vi "MIMIC Commands Rev 2.vi"(6 "MIMIC HOST COMMAND":T2(ring)=enum."Read Serial Number", 8 "Input String Data Array":string[](array[string])=["1"], 9 "HWHSflag":bool, 10 "wait (ms)":u32=500, 11 "VISA resource name":refnum<visa-resource-name>="COM5") -> (0 "error out":errorcluster={"status"=FALSE, "code"=1073676294, "source"="VISA Read in MIMIC RecvCommand.vi->MIMIC Commands Rev 2.vi"}, 1 "Receive_buffer":u8[](array[numeric]), 2 "Receive_Unpacked_Data":T1)   [LabVIEW 2014]
panel:
  out "Array":u8[](array[numeric])
  out "TimeToDecode":u16
  out "VISA resource name OUT":refnum<visa-resource-name>="COM5"
  out "hex integer string":string[](array[string])=["4", "D0", "0", "0", "FF", "2C"]
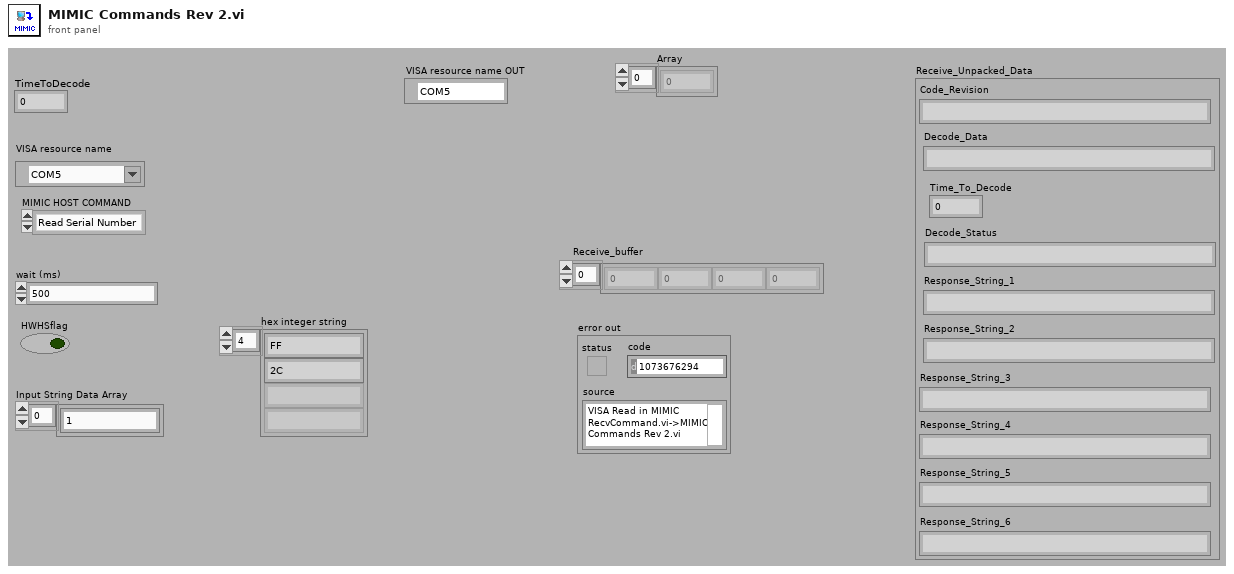
[diagram p1: front panel]
types:
  T1 = cluster{"Code_Revision":string, "Decode_Data":string, "Decode_Status":string, "Response_String_1":string, "Response_String_2":string, "Response_String_3":string, "Response_String_4":string, "Response_String_5":string, "Response_String_6":string, "Time_To_Decode":u16}
  T2 = enum16{"Enter FAT", "Beeper Control", "LED Off", "LED On", "Image Mode", "Start Session", "Stop Session", "Change Buadrate", "Auto Exposure", "Set Manual Exposure", "Read BT Address", "Store BT Address", "Pairing Command", "Query Paired Address", "Pairing Status", "Un-Pairing", "Set Illumination", "Trigger", "Set Defaults", "Imager Time To Decode Test", "Battery Off", "Battery Charge Control", "Read Battery Voltage", "Read Battery Temperature", "Software Version", "Store Feature Set", "Read Feature Set", "Store Model Number", "Read Model Number", "Store Manufacturing Date", "Read Manufacturing Date", "Store Service Date", "Read Service Date", "Store Serial Number", "Read Serial Number", "Exit FAT"}
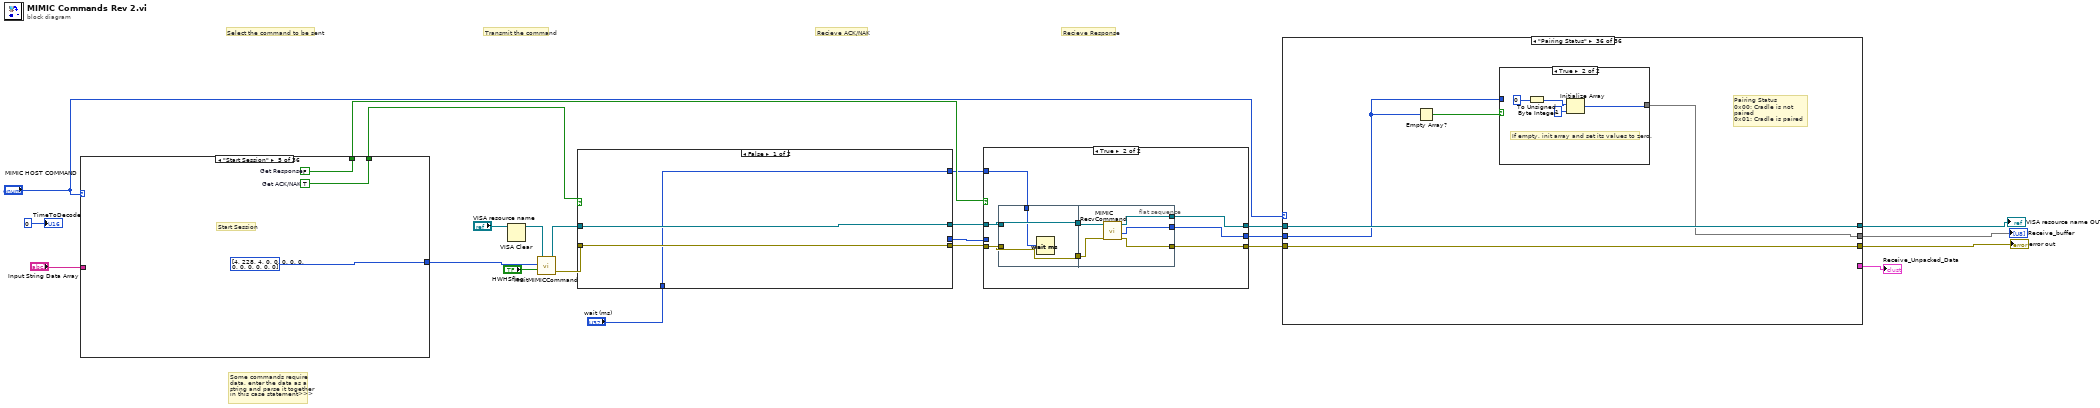
[diagram p0: block diagram]
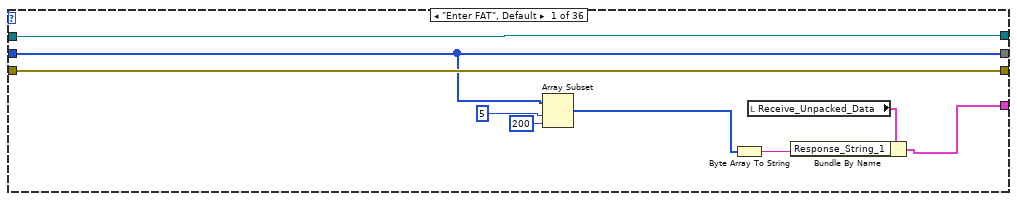
[diagram p2: hidden frame]
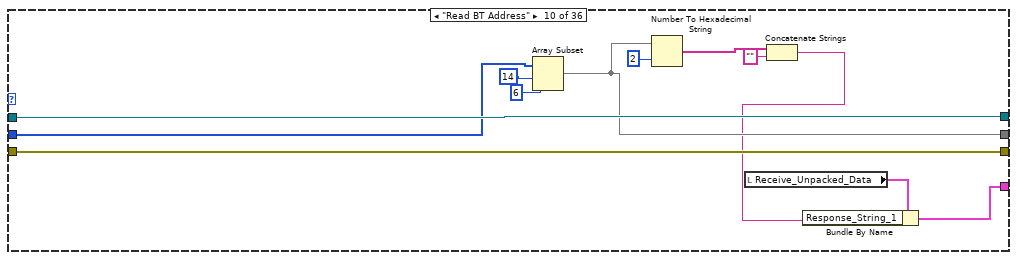
[diagram p11: hidden frame]
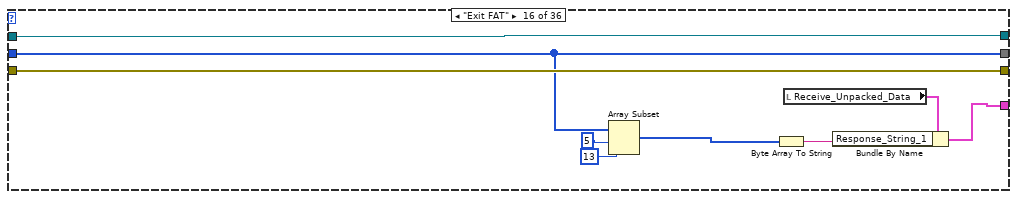
[diagram p17: hidden frame]
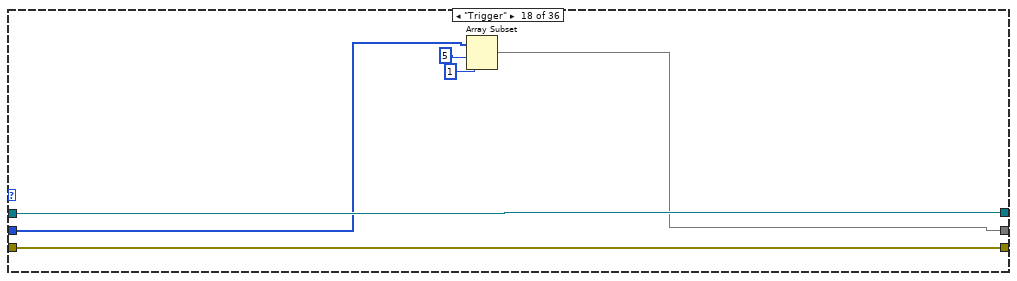
[diagram p19: hidden frame]
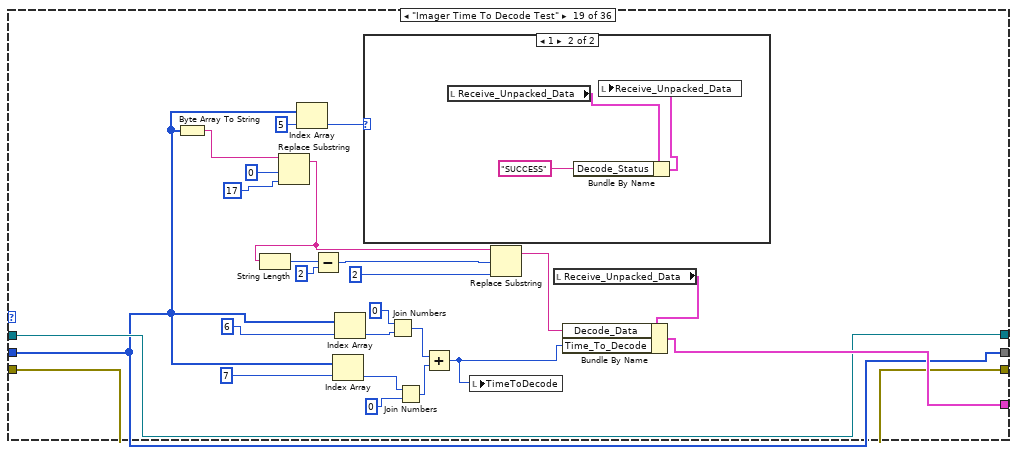
[diagram p20: hidden frame]
diagram:
  # "Transmit the command"
  # "Recieve Response"
  # "Recieve ACK/NAK"
  # "Select the command to be sent"
  # "Some commands require\ndata, enter the data as a\nstring and parse it together\nin this case statement>>>"
  n1 = case shown="\"Start Session\"" "MIMIC HOST COMMAND" {
    tunnel: "Input String Data Array" -> [w32 w33 _ w44 _ _ _ w62 w78 w88 w101 _ _ _ _ _ w125 _ _ _ w145 _ _ _ w161 _ w173 _ _ _ w199 _ w211 _ _ _]
    tunnel: [w26 w37 u8[] [5, 161, 4, 128, 16, 0, 0, 0, 0, 0, 0, 0, 0, 0] w45 u8[] [4, 228, 4, 0, 0, 0, 0, 0, 0, 0, 0, 0, 0, 0] u8[] [4, 228, 4, 0, 0, 0, 0, 0, 0, 0, 0, 0, 0, 0] u8[] [7, 215, 4, 0, 4, 11, 0, 255, 15, 0, 0, 0, 0, 0] w63 w72 w86 w100 u8[] [16, 161, 4, 128, 16, 0, 0, 0, 0, 0, 0, 0, 0, 0] u8[] [5, 161, 4, 128, 16, 0, 0, 0, 0, 0, 0, 0, 0, 0] u8[] [4, 200, 4, 128, 0, 0, 0, 0, 0, 0, 0, 0, 0, 0] u8[] [5, 161, 4, 128, 25, 0, 0, 0, 0, 0, 0, 0, 0, 0] u8[] [7, 161, 4, 128, 66, 2, 29, 0, 0, 0, 0, 0, 0, 0] w124 u8[] [6, 161, 4, 128, 45, 2, 0, 0, 0, 0, 0, 0, 0, 0] u8[] [7, 161, 4, 128, 48, 19, 136, 0, 0, 0, 0, 0, 0, 0] u8[] [5, 161, 4, 128, 60, 0, 0, 0, 0, 0, 0, 0, 0, 0] w144 u8[] [7, 161, 4, 128, 66, 117, 48, 0, 0, 0, 0, 0, 0, 0] u8[] [7, 161, 4, 128, 66, 117, 49, 0, 0, 0, 0, 0, 0, 0] u8[] [7, 161, 4, 128, 66, 78, 41, 0, 0, 0, 0, 0, 0, 0] w165 u8[] [7, 161, 4, 128, 66, 2, 194, 0, 0, 0, 0, 0, 0, 0] w178 u8[] [7, 161, 4, 128, 66, 2, 21, 0, 0, 0, 0, 0, 0, 0] w192 u8[] [7, 161, 4, 128, 66, 2, 23, 0, 0, 0, 0, 0, 0, 0] w204 u8[] [7, 161, 4, 128, 66, 2, 24, 0, 0, 0, 0, 0, 0, 0] w216 u8[] [7, 161, 4, 128, 66, 2, 22, 0, 0, 0, 0, 0, 0, 0] u8[] [5, 161, 4, 128, 54, 254, 160, 0, 0, 0, 0, 0, 0, 0] u8[] [5, 161, 4, 128, 84, 0, 0, 0, 0, 0, 0, 0, 0, 0]] -> w18
    tunnel: [w25 w35 w42 w46 w54 w57 w59 w64 w79 w89 w107 w110 w112 w115 w119 w123 w127 w134 w138 w141 w142 w153 w156 w158 w168 w171 w177 w182 w191 w196 w203 w207 w214 w219 w223 w227] -> w20
    tunnel: [w24 w36 w41 w47 w55 w58 w60 w65 w80 w90 w108 w111 w113 w116 w118 w122 w126 w135 w137 w140 w143 w152 w155 w157 w167 w170 w176 w183 w190 w195 w202 w208 w215 w220 w222 w226] -> w22
    frame "LED On" {
      w25 = FALSE  # Get Response
      w24 = TRUE  # Get ACK/NAK
      # "LED data Byte"
      n2 = Index Array(array=w32, index=0) -> (element=w31:string)
      n3 = Decimal String To Number(string=w31) -> (number=w30:i32)  [unwired: 2 in, 1 out]
      n4 = Replace Array Subset(array=u8[] [5, 231, 4, 128, 1, 0, 0, 0, 0, 0, 0, 0, 0, 0], new element=w30, index=4) -> (w26:u8[])
    }
    frame "Beeper Control" {
      w35 = FALSE  # Get Response
      w36 = FALSE  # Get ACK/NAK
      # "Beeper data Byte"
      n5 = Decimal String To Number(string=w33, offset=0) -> (number=w40:i32[])  [unwired: 1 in, 1 out]
      n6 = Replace Array Subset(array=u8[] [5, 230, 4, 128, 0, 0, 0, 0, 0, 0, 0, 0, 0, 0], new element=w40, index=4) -> (w37:u8[])
    }
    frame "Enter FAT" {
      w42 = TRUE  # Get Response
      w41 = TRUE  # Get ACK/NAK
      # "Enter FAT command:\n0x05:0xA1:0x40:0x80:0x10"
    }
    frame "Image Mode" {
      w46 = FALSE  # Get Response
      w47 = TRUE  # Get ACK/NAK
      # "Image Mode Byte:\n00: Decode\n01: SnapShot\n02: Video\n03: Last Decode\n04: las No Decode"
      n7 = Index Array(array=w44, index=0) -> (element=w52:string)
      n8 = Decimal String To Number(string=w52) -> (number=w51:i32)  [unwired: 2 in, 1 out]
      n9 = Replace Array Subset(array=u8[] [5, 247, 4, 128, 0, 0, 0, 0, 0, 0, 0, 0, 0, 0], new element=w51, index=4) -> (w45:u8[])
    }
    frame "Start Session" {
      w54 = FALSE  # Get Response
      w55 = TRUE  # Get ACK/NAK
      # "Start Session"
    }
    frame "Stop Session" {
      w57 = FALSE  # Get Response
      w58 = TRUE  # Get ACK/NAK
      # "Start Session"
    }
    frame "Change Buadrate" {
      w59 = FALSE  # Get Response
      w60 = FALSE  # Get ACK/NAK
      # "Enter FAT command:\n06: 9600\n08: 38400\n0A: 57600\n0B:115200\n0C:230400"
    }
    frame "Auto Exposure" {
      w64 = FALSE  # Get Response
      w65 = TRUE  # Get ACK/NAK
      # "Auto Exposure:\n00:Disabled\n01: Enabled"
      n10 = Index Array(array=w62, index=0) -> (element=w70:string)
      n11 = Decimal String To Number(string=w70) -> (number=w69:i32)  [unwired: 2 in, 1 out]
      n12 = Replace Array Subset(array=u8[] [8, 198, 4, 0, 255, 240, 41, 0, 0, 0, 0, 0, 0, 0], new element=w69, index=7) -> (w63:u8[])
    }
    frame "Set Manual Exposure" {
      w79 = FALSE  # Get Response
      w80 = TRUE  # Get ACK/NAK
      # "Image Mode Byte:\n00: Decode\n01: SnapShot\n02: Video\n03: Last Decode\n04: las No Decode"
      n13 = Index Array(array=w78, index=0) -> (element=w84:string)
      n14 = Decimal String To Number(string=w84, default (0L)=u16 0 ("default (0 I32)")) -> (number=w77:u16)  [unwired: 1 in, 1 out]
      n15 = Split Number(x=w77) -> (hi(x)=w75:u8, lo(x)=w74:u8)
      n16 = Replace Array Subset(array=u8[] [10, 198, 4, 0, 255, 244, 241, 55, 0, 0, 0, 0, 0, 0], new element=w75, index=8) -> (w71:u8[])
      n17 = Replace Array Subset(array=w71, new element=w74, index=9) -> (w72:u8[])
    }
    frame "Store BT Address" {
      w89 = FALSE  # Get Response
      w90 = TRUE  # Get ACK/NAK
      # "Store BT command:\n0x16, 0xA1, 0x04, 0x80, 0x45, 0x02, 0x1D, 0x41, 0x07, 0x42, 0x00, 0x06, 0x00, 0x00, \n\t\t\t\t\t\t\t\t\t\t0x00, 0x00, 0x00, 0x00, 0x00, 0x00,0x00, 0x00, 0xFF, 0xFF};"
      n18 = for {
        N: 6 -> [_]
        tunnel: w88 -> [w99]
        tunnel: [w94] -> w86
        i -> [w96]
        n19 = Index Array(array=w99, index=w96) -> (element=w93:string)
        n20 = Add(x=14 ("index"), y=w96) -> (x+y=w97:i32)
        n21 = Hexadecimal String To Number(string=w93, offset=0) -> (number=w91:u32)  [unwired: 1 in, 1 out]
        n22 = local read "Array"() -> (w95:u8[])
        n23 = Replace Array Subset(array=w95, new element=w91, index=w97) -> (w94:u8[])
        n24 = local write "Array"(w94) -> ()
      }
      "Array" <- u8[] [22, 161, 4, 128, 69, 2, 29, 65, 7, 66, 0, 6, 0, 0, 0, 0, 0, 0, 0, 0, 255, 255, 255, 0, 0, 0]
    }
    frame "Pairing Command" {
      w107 = TRUE  # Get Response
      w108 = FALSE  # Get ACK/NAK
      # "Pairing  command:\n10 9E 04 80 00 00 02 03 06 08  01 0B 03 00 0F 0F FE 8E"
      n25 = Index Array(array=w101, index=0) -> (element=w105:string)
      n26 = String To Byte Array(string=w105) -> (unsigned byte array=w103:u8[])
      n27 = Replace Array Subset(array=u8[] [16, 158, 4, 128, 0, 0, 0, 0, 0, 8, 1, 11, 3, 0, 15, 15], new element=w103, index=4) -> (w100:u8[])
    }
    frame "Un-Pairing" {
      w110 = TRUE  # Get Response
      w111 = FALSE  # Get ACK/NAK
      # "Enter FAT command:\n0x05:0xA1:0x40:0x80:0x10"
    }
    frame "Set Illumination" {
      w112 = TRUE  # Get Response
      w113 = FALSE  # Get ACK/NAK
      # "Enter FAT command:\n0x05:0xA1:0x40:0x80:0x10"
    }
    frame "Set Defaults" {
      w115 = FALSE  # Get Response
      w116 = TRUE  # Get ACK/NAK
    }
    frame "Exit FAT" {
      w119 = TRUE  # Get Response
      w118 = TRUE  # Get ACK/NAK
    }
    frame "Read BT Address" {
      w123 = TRUE  # Get Response
      w122 = FALSE  # Get ACK/NAK
    }
    frame "LED Off" {
      w127 = FALSE  # Get Response
      w126 = TRUE  # Get ACK/NAK
      # "LED data Byte"
      n28 = Index Array(array=w125, index=0) -> (element=w132:string)
      n29 = Decimal String To Number(string=w132) -> (number=w131:i32)  [unwired: 2 in, 1 out]
      n30 = Replace Array Subset(array=u8[] [5, 232, 4, 128, 1, 0, 0, 0, 0, 0, 0, 0, 0, 0], new element=w131, index=4) -> (w124:u8[])
    }
    frame "Trigger" {
      w134 = TRUE  # Get Response
      w135 = TRUE  # Get ACK/NAK
    }
    frame "Imager Time To Decode Test" {
      w138 = TRUE  # Get Response
      w137 = TRUE  # Get ACK/NAK
      # "Start Session"
    }
    frame "Battery Off" {
      w141 = FALSE  # Get Response
      w140 = TRUE  # Get ACK/NAK
      # "Enter FAT command:\n0x05:0xA1:0x40:0x80:0x10"
    }
    frame "Battery Charge Control" {
      w142 = FALSE  # Get Response
      w143 = TRUE  # Get ACK/NAK
      # "Battery Charge\n0x06, 0xA1, 0x04, 0x80, 0x3D\n0x00: Disable charging of battery\n0x01: Enable charging of battery\n0x02: Enable Slow charge (Hammer)"
      n31 = Index Array(array=w145, index=0) -> (element=w150:string)
      n32 = Decimal String To Number(string=w150) -> (number=w149:i32)  [unwired: 2 in, 1 out]
      n33 = Replace Array Subset(array=u8[] [6, 161, 4, 128, 61, 0, 0, 0, 0, 0, 0, 0, 0, 0], new element=w149, index=5) -> (w144:u8[])
    }
    frame "Read Battery Voltage" {
      w153 = TRUE  # Get Response
      w152 = FALSE  # Get ACK/NAK
      # "Read Battery Voltage command:\n0x07:0xA1:0x04:0x80:0x42:0x75:0x30"
    }
    frame "Read Battery Temperature" {
      w156 = TRUE  # Get Response
      w155 = FALSE  # Get ACK/NAK
      # "Read Battery Temperature command:\n0x07:0xA1:0x04:0x80:0x42:0x75:0x31"
    }
    frame "Software Version" {
      w158 = TRUE  # Get Response
      w157 = TRUE  # Get ACK/NAK
      # "Software Version command:\n\"0x07, 0xA1, 0x04, 0x80, 0x42, 0x4E, 0x29,\""
    }
    frame "Store Feature Set" {
      w168 = FALSE  # Get Response
      w167 = TRUE  # Get ACK/NAK
      # "Store Feature Set command:\n\"0x0A, 0xA1, 0x04, 0x80, 0x45, 0x02, 0xC2, 0x42, 0x07,\n0xFF,//Feature Set Value \n0x00, 0x00}; //checksum\""
      n34 = Index Array(array=w161, index=0) -> (element=w163:string)
      n35 = String To Byte Array(string=w163) -> (unsigned byte array=w160:u8[])
      n36 = Replace Array Subset(array=u8[] [10, 161, 4, 128, 69, 2, 194, 66, 7, 0, 0, 0, 0, 0], new element=w160, index=9) -> (w165:u8[])
    }
    frame "Read Feature Set" {
      w171 = TRUE  # Get Response
      w170 = FALSE  # Get ACK/NAK
      # "Read Feature Set command:\n0x07, 0xA1, 0x04, 0x80, 0x42, 0x02, 0xC2,"
    }
    frame "Store Model Number" {
      w177 = FALSE  # Get Response
      w176 = TRUE  # Get ACK/NAK
      # "StoreModel Number command:\n0x20, 0xA1, 0x04, 0x80, 0x45, 0x02, 0x15, 0x53, 0x07, 0x00, 0x12, 0x00, 0x00,\n\t\t\t\t\t\t\t\t\t\t0x00, 0x00, 0x00, 0x00, 0x00, 0x00, 0x00, 0x00, 0x00,\n\t\t\t\t\t\t\t\t\t\t0x00, 0x00, 0x00, 0x00, 0x00, 0x00, 0x00, 0x00, 0x00,\n\t\t\t\t\t\t\t\t\t\t0x00"
      n37 = Index Array(array=w173, index=0) -> (element=w174:string)
      n38 = String To Byte Array(string=w174) -> (unsigned byte array=w175:u8[])
      n39 = Replace Array Subset(array=u8[] [32, 161, 4, 128, 69, 2, 21, 83, 7, 0, 18, 0, 0, 0, 0, 0, 0, 0, 0, 0, 0, 0, 0, 0, 0, 0, 0, 0, 0, 0, 0, 0, 0], new element=w175, index=13) -> (w178:u8[])
    }
    frame "Read Model Number" {
      w182 = TRUE  # Get Response
      w183 = TRUE  # Get ACK/NAK
      # "ReadModel Number command:\n0x07, 0xA1, 0x04, 0x80, 0x42, 0x02, 0x15,"
    }
    frame "Store Manufacturing Date" {
      w191 = FALSE  # Get Response
      w190 = TRUE  # Get ACK/NAK
      # "Store Manufacturing Date command:\n0x15, 0xA1, 0x04, 0x80, 0x45, 0x02, 0x17, 0x53, 0x07, 0x00, 0x07, 0x00, 0x00,\n\t\t\t\t\t\t\t\t\t\t0x00, 0x00, 0x00, 0x00, 0x00, 0x00, 0x00,\n\t\t\t\t\t\t\t\t\t\t0x00"
      n40 = Get Date/Time In Seconds() -> (seconds since 1Jan1904=w189:timestamp)
      n41 = Format Date/Time String(time format string (%c)="%d%b%y", seconds (now)=w189, UTC format=FALSE) -> (date/time string=w185:string)
      n42 = To Upper Case(1:w185) -> (0:w184:string)
      n43 = String To Byte Array(string=w184) -> (unsigned byte array=w186:u8[])
      n44 = Replace Array Subset(array=u8[] [21, 161, 4, 128, 69, 2, 23, 83, 7, 0, 7, 0, 0, 0, 0, 0, 0, 0, 0, 0, 0, 0], new element=w186, index=13) -> (w192:u8[])
    }
    frame "Read Manufacturing Date" {
      w196 = TRUE  # Get Response
      w195 = TRUE  # Get ACK/NAK
      # "Read Feature Set command:\n0x07, 0xA1, 0x04, 0x80, 0x42, 0x02, 0x17,"
    }
    frame "Store Service Date" {
      w203 = FALSE  # Get Response
      w202 = TRUE  # Get ACK/NAK
      # "StoreService Date command:\n0x15, 0xA1, 0x04, 0x80, 0x45, 0x02, 0x18, 0x53, 0x07, 0x00, 0x07, 0x00, 0x00,\n\t\t\t\t\t\t\t\t\t\t0x00, 0x00, 0x00, 0x00, 0x00, 0x00, 0x00,\n\t\t\t\t\t\t\t\t\t\t0x00"
      n45 = Index Array(array=w199, index=0) -> (element=w201:string)
      n46 = String To Byte Array(string=w201) -> (unsigned byte array=w198:u8[])
      n47 = Replace Array Subset(array=u8[] [21, 161, 4, 128, 69, 2, 24, 83, 7, 0, 7, 0, 0, 0, 0, 0, 0, 0, 0, 0, 0, 0], new element=w198, index=13) -> (w204:u8[])
    }
    frame "Read Service Date" {
      w207 = TRUE  # Get Response
      w208 = TRUE  # Get ACK/NAK
      # "Read Service Date command:\n0x07, 0xA1, 0x04, 0x80, 0x42, 0x02, 0x18,"
    }
    frame "Store Serial Number" {
      w214 = FALSE  # Get Response
      w215 = TRUE  # Get ACK/NAK
      # "Store Serial Number command:\n0x1E, 0xA1, 0x04, 0x80, 0x45, 0x02, 0x16, 0x53, 0x07, 0x00, 0x10, 0x00, 0x00,\n\t\t\t\t\t\t\t\t\t\t0x00, 0x00, 0x00, 0x00, 0x00, 0x00, 0x00, 0x00,\n\t\t\t\t\t\t\t\t\t\t0x00, 0x00, 0x00, 0x00, 0x00, 0x00, 0x00, 0x00,\n\t\t\t\t\t\t\t\t\t\t0x00"
      n48 = Index Array(array=w211, index=0) -> (element=w213:string)
      n49 = String To Byte Array(string=w213) -> (unsigned byte array=w210:u8[])
      n50 = Replace Array Subset(array=u8[] [30, 161, 4, 128, 69, 2, 22, 83, 7, 0, 16, 0, 0, 0, 0, 0, 0, 0, 0, 0, 0, 0, 0, 0, 0, 0, 0, 0, 0, 0, 0, 0, 0], new element=w210, index=13) -> (w216:u8[])
    }
    frame "Read Serial Number" {
      w219 = TRUE  # Get Response
      w220 = TRUE  # Get ACK/NAK
      # "Read Serial Number command:\n0x07, 0xA1, 0x04, 0x80, 0x42, 0x02, 0x16,"
    }
    frame "Pairing Status" {
      w223 = TRUE  # Get Response
      w222 = FALSE  # Get ACK/NAK
      # "Read Serial Number command:\n0x05, 0xA1, 0x04, 0x80, 0x36, 0xFE, 0xA0,"
    }
    frame "Query Paired Address" {
      w227 = TRUE  # Get Response
      w226 = FALSE  # Get ACK/NAK
      # "Read Serial Number command:\n0x05, 0xA1, 0x04, 0x80, 0x54,"
    }
  }
  n51 = VISA Clear(VISA resource name="VISA resource name") -> (VISA resource name out=w8:refnum<visa-resource-name>)  [unwired: 1 in, 1 out]
  n52 = call "XmitMIMICCommand.vi"("HWHSflag"="HWHSflag", "Command array"=w18, "VISA resource name"=w8) -> ("error out"=w16:errorcluster, "VISA resource name Out"=w15:refnum<visa-resource-name>)  [unwired: 1 in]
  n53 = case shown="False" w22 {
    tunnel: [w230 w234] -> w21
    tunnel: w16 -> [w230 w239]
    tunnel: w15 -> [w229 w237]
    tunnel: [w229 w235] -> w19
    tunnel: [_ w233] -> w10
    tunnel: [w228 w232] -> w7
    tunnel: "wait (ms)" -> [w228 w231]
    frame False {
    }
    frame True {
      # "NEED TO CHECK ACK"
      n54 = flat-sequence {
        tunnel: w239 -> [w242]
        tunnel: [w242] -> w238
        tunnel: w237 -> [w241]
        tunnel: [w241] -> w236
        tunnel: [w240] -> w232
        tunnel: w231 -> [w240]
        tunnel: w238 -> [w247]
        tunnel: w236 -> [w246]
        tunnel: [w245] -> w235
        tunnel: [w244] -> w234
        tunnel: [w243] -> w233
        frame #0 {
          n55 = Wait (ms)(milliseconds to wait=w240) -> ()  [unwired: 1 out]
        }
        frame #1 {
          n56 = call "MIMIC RecvCommand.vi"("error in"=w247, "VISA resource name"=w246) -> ("error out"=w244:errorcluster, "Receive_buffer"=w243:u8[], "VISA resource name OUT"=w245:refnum<visa-resource-name>)  [unwired: 2 in, 1 out]
          n57 = Number To Hexadecimal String(2:w243) -> (0:→"hex integer string":string[])  [unwired: 1 in]
        }
      }
    }
  }
  n58 = case shown="True" w20 {
    tunnel: [w251 w258] -> w11
    tunnel: w21 -> [w251 w253]
    tunnel: w19 -> [w250 w255]
    tunnel: [w249 w259] -> w12
    tunnel: [w250 w257] -> w13
    tunnel: w10 -> [w249 _]
    tunnel: w7 -> [_ w252]
    frame False {
    }
    frame True {
      n59 = flat-sequence {
        tunnel: [w262] -> w256
        tunnel: w255 -> [w262]
        tunnel: [w261] -> w254
        tunnel: w253 -> [w261]
        tunnel: w252 -> [w260]
        tunnel: [w267] -> w259
        tunnel: [w266] -> w258
        tunnel: [w265] -> w257
        tunnel: w256 -> [w263]
        tunnel: w254 -> [w264]
        frame #0 {
          n60 = Wait (ms)(milliseconds to wait=w260) -> ()  [unwired: 1 out]
        }
        frame #1 {
          n61 = call "MIMIC RecvCommand.vi"("error in"=w264, "VISA resource name"=w263) -> ("error out"=w266:errorcluster, "Receive_buffer"=w267:u8[], "VISA resource name OUT"=w265:refnum<visa-resource-name>)  [unwired: 2 in, 1 out]
        }
      }
    }
  }
  n62 = case shown="\"Pairing Status\"" "MIMIC HOST COMMAND" {
    tunnel: w13 -> [w275 w279 w282 w285 w288 w291 w294 w297 w300 w312 w315 w318 w321 w324 w327 w336 w339 w345 w356 w379 w382 w388 w390 w400 w406 w409 w413 w423 w434 w442 w445 w454 w456 w467 w478 w483]
    tunnel: [w275 w279 w282 w285 w288 w291 w294 w297 w300 w312 w315 w318 w321 w324 w327 w336 w339 w345 w356 w379 w382 w388 w390 w400 w406 w409 w413 w423 w434 w442 w445 w454 w456 w467 w478 w483] -> w5
    tunnel: w12 -> [w271 w278 w281 w284 w287 w290 w293 w296 w299 w310 w314 w317 w320 w323 w326 w328 w338 w341 w354 w378 w381 w384 w392 w401 w405 w410 w414 w420 w433 w439 w444 w451 w457 w463 w471 w480]
    tunnel: [w271 w278 w281 w284 w287 w290 w293 w296 w299 w305 w314 w317 w320 w323 w326 w328 w338 w340 w354 w378 w381 w383 w391 w398 w405 w407 w414 w418 w433 w436 w444 w449 w457 w459 w469 w482] -> w4
    tunnel: w11 -> [w276 w277 w280 w283 w286 w289 w292 w295 w298 w311 w313 w316 w319 w322 w325 w335 w337 w344 w357 w377 w380 w387 w389 w399 w404 w408 w415 w424 w432 w443 w446 w455 w458 w466 w479 w484]
    tunnel: [w276 w277 w280 w283 w286 w289 w292 w295 w298 w311 w313 w316 w319 w322 w325 w335 w337 w344 w357 w377 w380 w387 w389 w399 w404 w408 w415 w424 w432 w443 w446 w455 w458 w466 w479 w484] -> w3
    tunnel: [w273 _ _ _ _ _ _ _ _ w306 _ _ _ _ _ w332 _ _ w359 _ _ _ _ w395 _ _ _ w416 w426 w437 _ w447 _ w461 w470 _] -> w1
    frame "Enter FAT", Default {
      n63 = Array Subset(array=w271, index=5, length=200) -> (w270:u8[])
      n64 = Byte Array To String(unsigned byte array=w270) -> (string=w274:string)
      n65 = local read "Receive_Unpacked_Data"() -> (w272:T1)
      n66 = Bundle By Name(cluster=w272, "Response_String_1"=w274) -> (w273:T1)
    }
    frame "Beeper Control" {
    }
    frame "LED On" {
    }
    frame "Image Mode" {
    }
    frame "Start Session" {
    }
    frame "Stop Session" {
    }
    frame "Change Buadrate" {
    }
    frame "Auto Exposure" {
    }
    frame "Set Manual Exposure" {
    }
    frame "Read BT Address" {
      n67 = Array Subset(array=w310, index=14, length=6) -> (w305:u8[])
      n68 = Number To Hexadecimal String(1:i16 2 ("width (-)"), 2:w305) -> (0:w303:string[])
      n69 = local read "Receive_Unpacked_Data"() -> (w307:T1)
      n70 = Concatenate Strings(w303, "" ("string")) -> (w302:string)
      n71 = Bundle By Name(cluster=w307, "Response_String_1"=w302) -> (w306:T1)
    }
    frame "Store BT Address" {
    }
    frame "Pairing Command" {
    }
    frame "Un-Pairing" {
    }
    frame "Set Illumination" {
    }
    frame "Set Defaults" {
    }
    frame "Exit FAT" {
      n72 = Array Subset(array=w328, index=5, length=13) -> (w329:u8[])
      n73 = Byte Array To String(unsigned byte array=w329) -> (string=w334:string)
      n74 = local read "Receive_Unpacked_Data"() -> (w333:T1)
      n75 = Bundle By Name(cluster=w333, "Response_String_1"=w334) -> (w332:T1)
    }
    frame "LED Off" {
    }
    frame "Trigger" {
      n76 = Array Subset(array=w341, index=5, length=1) -> (w340:u8[])
    }
    frame "Imager Time To Decode Test" {
      n77 = Byte Array To String(unsigned byte array=w354) -> (string=w370:string)
      n78 = Replace Substring(2:17 ("length (len. of substring)"), 3:0 ("offset (0)"), 5:w370) -> (1:w365:string)  [unwired: 1 in, 1 out]
      n79 = String Length(string=w365) -> (length=w364:i32)
      n80 = Index Array(array=w354, index=5) -> (element=w367:u8)
      n81 = Subtract(x=w364, y=2) -> (x-y=w362:i32)
      n82 = Index Array(array=w354, index=7 ("length")) -> (element=w349:u8)
      n83 = Index Array(array=w354, index=6) -> (element=w352:u8)
      n84 = case shown="1" w367 {
        frame 0, Default {
          n85 = local read "Receive_Unpacked_Data"() -> (w371:T1)
          n86 = Bundle By Name(cluster=w371, "Decode_Status"="No Decode" ("Decode_Data")) -> (w372:T1)
          n87 = local write "Receive_Unpacked_Data"(w372) -> ()
        }
        frame 1 {
          n88 = local read "Receive_Unpacked_Data"() -> (w375:T1)
          n89 = Bundle By Name(cluster=w375, "Decode_Status"="SUCCESS" ("Decode_Data")) -> (w374:T1)
          n90 = local write "Receive_Unpacked_Data"(w374) -> ()
        }
      }
      n91 = Join Numbers(hi=u8 0, lo=w352) -> ((hi.lo)=w347:u16)
      n92 = Join Numbers(hi=w349, lo=u8 0 ("hi")) -> ((hi.lo)=w348:u16)
      n93 = Add(x=w347, y=w348) -> (x+y=w346:u16)
      n94 = local write "TimeToDecode"(w346) -> ()
      n95 = Replace Substring(2:2 ("length (len. of substring)"), 3:w362, 5:w365) -> (1:w360:string)  [unwired: 1 in, 1 out]
      n96 = local read "Receive_Unpacked_Data"() -> (w358:T1)
      n97 = Bundle By Name(cluster=w358, "Decode_Data"=w360, "Time_To_Decode"=w346) -> (w359:T1)
    }
    frame "Battery Off" {
    }
    frame "Battery Charge Control" {
    }
    frame "Read Battery Voltage" {
      # "Voltage (MSB_LSB *.0006*2)"
      # "RESPONSE\nLength Byte:\t0x0D\nOpcode Byte:\t0x21\nSource Byte:\t0x00\nStatus Byte:\t0x80\nSub-opcode Byte:\t0x42\nData Byte 1:\t0x75: Attribute MSB\nData Byte 2:\t0x30: Attribute LSB\nData Byte 3:\t0x57: Attribute is Word ('W') value\nData Byte 4:\t0x01\nData Byte 5:\t0xXX: Battery Voltage MSB\nData Byte 6:\t0xXX: Battery Voltage LSB\nData Byte 7:\t0xFF: Packet Termination\nData Byte 8:\t0xFF: Packet Termination\nChecksum High Byte:\t0xXX\nChecksum Low Byte:\t0xXX"
      n98 = Array Subset(array=w384, index=0, length=15) -> (w383:u8[])
    }
    frame "Read Battery Temperature" {
      # "RESPONSE\nLength Byte:\t0x0D\nOpcode Byte:\t0x21\nSource Byte:\t0x00\nStatus Byte:\t0x80\nSub-opcode Byte:\t0x42\nData Byte 1:\t0x75: Attribute MSB\nData Byte 2:\t0x31: Attribute LSB\nData Byte 3:\t0x57: Attribute is Word ('W') value\nData Byte 4:\t0x01\nData Byte 5:\t0xXX: Battery Temperature MSB\nData Byte 6:\t0xXX: Battery Temperature LSB\nData Byte 7:\t0xFF: Packet Termination\nData Byte 8:\t0xFF: Packet Termination\nChecksum High Byte:\t0xXX\nChecksum Low Byte:\t0xXX"
      n99 = Array Subset(array=w392, index=0, length=15) -> (w391:u8[])
    }
    frame "Software Version" {
      n100 = Array Subset(array=w401, index=13, length=18) -> (w398:u8[])
      n101 = Byte Array To String(unsigned byte array=w398) -> (string=w397:string)
      n102 = local read "Receive_Unpacked_Data"() -> (w396:T1)
      n103 = Bundle By Name(cluster=w396, "Code_Revision"=w397) -> (w395:T1)
    }
    frame "Store Feature Set" {
    }
    frame "Read Feature Set" {
      # "Feature Set Responce:\n0x0C, 0x21, 0x00, 0x00, 0x42, 0x02, 0xC2,0x42,0x01,\n\t\t\t\t\t\t\t\t\t\t\t  \t\t\t  0xff, //FEATURE-SET\n\t\t\t\t\t\t\t\t\t\t\t\t\t\t  0xff,0xff, // packet termination\n\t\t\t\t\t\t\t\t\t\t\t\t\t\t  0x00, 0x00}; //checksum"
      n104 = Array Subset(array=w410, index=9, length=1) -> (w407:u8[])
    }
    frame "Store Model Number" {
    }
    frame "Read Model Number" {
      n105 = Array Subset(array=w420, index=13, length=18) -> (w418:u8[])
      n106 = Byte Array To String(unsigned byte array=w418) -> (string=w419:string)
      n107 = local read "Receive_Unpacked_Data"() -> (w417:T1)
      n108 = Bundle By Name(cluster=w417, "Response_String_1"=w419) -> (w416:T1)
    }
    frame "Store Manufacturing Date" {
      n109 = Get Date/Time In Seconds() -> (seconds since 1Jan1904=w431:timestamp)
      n110 = Format Date/Time String(time format string (%c)="%d%b%y", seconds (now)=w431, UTC format=FALSE) -> (date/time string=w428:string)
      n111 = To Upper Case(1:w428) -> (0:w425:string)
      n112 = local read "Receive_Unpacked_Data"() -> (w427:T1)
      n113 = Bundle By Name(cluster=w427, "Response_String_1"=w425) -> (w426:T1)
    }
    frame "Read Manufacturing Date" {
      n114 = Array Subset(array=w439, index=13, length=7) -> (w436:u8[])
      n115 = Byte Array To String(unsigned byte array=w436) -> (string=w438:string)
      n116 = local read "Receive_Unpacked_Data"() -> (w435:T1)
      n117 = Bundle By Name(cluster=w435, "Response_String_1"=w438) -> (w437:T1)
    }
    frame "Store Service Date" {
    }
    frame "Read Service Date" {
      n118 = Array Subset(array=w451, index=13, length=7) -> (w449:u8[])
      n119 = Byte Array To String(unsigned byte array=w449) -> (string=w450:string)
      n120 = local read "Receive_Unpacked_Data"() -> (w448:T1)
      n121 = Bundle By Name(cluster=w448, "Response_String_1"=w450) -> (w447:T1)
    }
    frame "Store Serial Number" {
    }
    frame "Read Serial Number" {
      n122 = Array Subset(array=w463, index=13, length=16) -> (w459:u8[])
      n123 = Byte Array To String(unsigned byte array=w459) -> (string=w462:string)
      n124 = local read "Receive_Unpacked_Data"() -> (w460:T1)
      n125 = Bundle By Name(cluster=w460, "Response_String_1"=w462) -> (w461:T1)
    }
    frame "Query Paired Address" {
      # "Cradle BT Address"
      # "Pair Status\n0x00: Unpaired \n0x01: Paired"
      n126 = Array Subset(array=w471, index=6, length=6) -> (w474:u8[])
      n127 = Array Subset(array=w471, index=5, length=1) -> (w469:u8[])
      n128 = local read "Receive_Unpacked_Data"() -> (w468:T1)
      n129 = Byte Array To String(unsigned byte array=w474) -> (string=w475:string)
      n130 = Bundle By Name(cluster=w468, "Response_String_1"=w475) -> (w470:T1)
    }
    frame "Pairing Status" {
      # "Pairing Status\n0x00: Cradle is not paired\n0x01: Cradle is paired"
      n131 = Empty Array?(array=w480) -> (empty?=w481:bool)
      n132 = case shown="True" w481 {
        tunnel: w480 -> [w486 _]
        tunnel: [w485 w492] -> w482
        frame False {
          n133 = Array Subset(array=w486, index=5, length=1) -> (w485:u8[])
        }
        frame True {
          # "If empty, init array and set its values to zero."
          n134 = To Unsigned Byte Integer(number=u8 0) -> (unsigned 8bit integer=w490:u8)
          n135 = Initialize Array(w490, 1 ("dimension size")) -> (w492:u8[])
        }
      }
    }
  }
  "error out" <- w3
  "Receive_buffer" <- w4
  "VISA resource name OUT" <- w5
  "Receive_Unpacked_Data" <- w1
  "TimeToDecode" <- u16 0 ("TimeToDecode")
